vi "Set SkipName.vi"(8 "error in (no error)":errorcluster, 10 "SkipName":bool, 11 "GetTypeAttributesVisitor.lvclass in":refnum<class "GetTypeAttributesVisitor.lvclass">) -> (0 "error out":errorcluster, 3 "GetTypeAttributesVisitor.lvclass out":refnum<class "GetTypeAttributesVisitor.lvclass">)   [LabVIEW 2020, in "Web Service Description.lvlib" / "GetTypeAttributesVisitor.lvclass"]
uses:
  <vilib>/AppBuilder/Engine/WebServiceDescription/GetTypeAttributesVisitor/GetTypeAttributesVisitor.lvclass
  <vilib>/AppBuilder/Engine/WebServiceDescription/GetTypeAttributesVisitor/GetTypeAttributesVisitor.lvclass/GetTypeAttributesVisitor.ctl
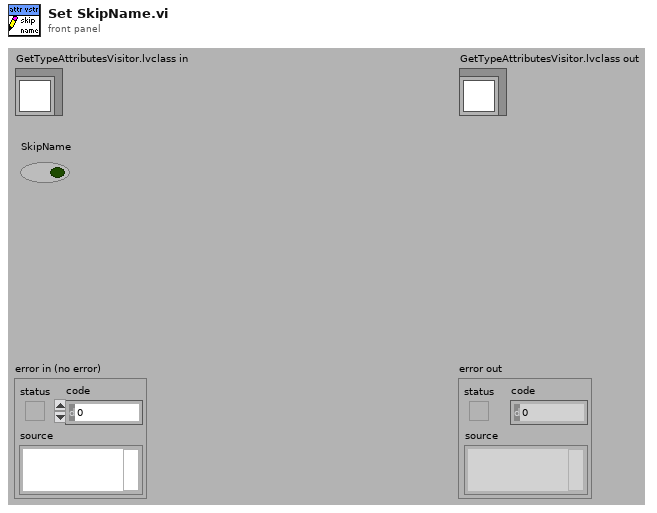
[diagram p1: front panel]
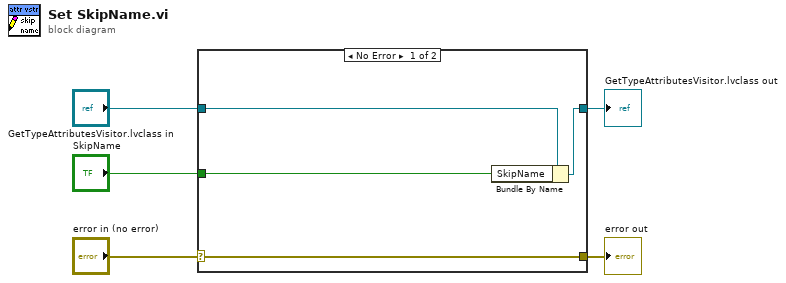
[diagram p0: block diagram]
diagram:
  n1 = case shown="No Error" "error in (no error)" {
    selector: "error in (no error)" -> [w9 w10]
    tunnel: [w9 w10] -> w4
    tunnel: [w7 w11] -> w2
    tunnel: "GetTypeAttributesVisitor.lvclass in" -> [w8 w11]
    tunnel: "SkipName" -> [w6 _]
    frame No Error {
      n2 = Bundle By Name(cluster=w8, "SkipName"=w6) -> (w7:refnum<class "GetTypeAttributesVisitor.lvclass">)
    }
    frame Error {
    }
  }
  "error out" <- w4
  "GetTypeAttributesVisitor.lvclass out" <- w2
